vi "Open LabVIEW Folder.vi"   [LabVIEW 2014]
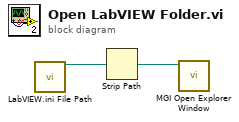
[diagram p0: block diagram]
diagram:
  n1 = call "LabVIEW.ini File Path.vi"() -> ("appended path"=w2:path)  [unwired: 19 in]
  n2 = Strip Path(path=w2) -> (stripped path=w1:path)  [unwired: 1 out]
  n3 = call <userlib>:"MGI Open Explorer Window.vi"("Directory or File"=w1) -> ()  [unwired: 10 in, 1 out]
